vi "Do_Multical.vi"(7 "Rig Name":string, 9 "Rig Gas Selector Ch":T1[](array[typedef]) {"Duty" format="%.0b"; "D" format="%#_5g"; "C" format="%#_5g"; "B" format="%#_5g"; "A" format="%#_5g"}, 10 "Cal Gas Selection":string[](array[string]), 11 "Calib Filepaths":path[](array[path])) -> (2 "Cal Data":dbl[][](array[numeric]), 3 "Ref Data":dbl[](array[numeric]))   [LabVIEW 2015]
doc: "Step through the Calibration Procedure:\n1. Prompt user to connect appropriate / expected Cal Gas\n2. Update \"Gas Selector\" ADAM Ch which points to the current Cal Gas ADAM Ch\n3. Wait for sample to reach FID and settle\n4. Get a calibration data point for each FID"
uses:
  ADAM Client/Sub VIs/ADAM Controls/Ch_description_ADAM.ctl
  ADAM Client/Sub VIs/ADAM Controls/Module_type_ADAM.ctl
  ADAM Client/Sub VIs/ADAM Controls/Function_ADAM.ctl
  ADAM Client/Sub VIs/ADAM Controls/Channel_State.ctl
  ADAM Client/Sub VIs/ADAM Controls/Calib_type_ADAM.ctl
  ADAM Client/Sub VIs/ADAM Controls/Address.ctl
panel:
  in  "Tab Control":enum32{"Input", "Output"}(tab)
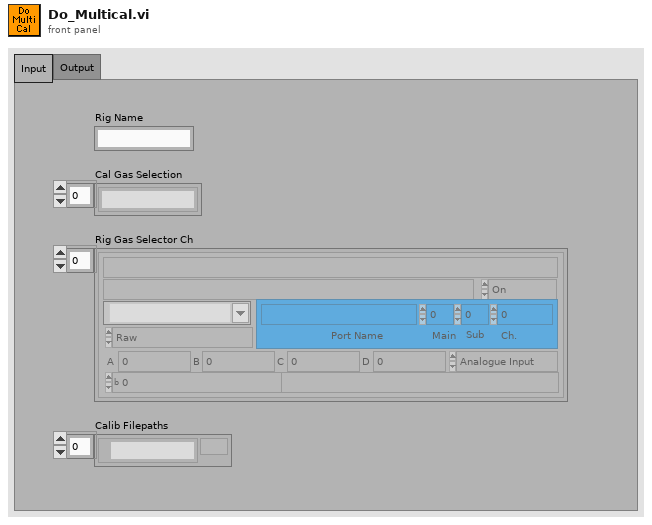
[diagram p1: front panel]
types:
  T1 = typedef "Ch_description_ADAM.ctl" = cluster{"Ch Name":string, "Type":T2, "Function":T3, "Ch State":T4, "Calibration type":T5, "A":dbl, "B":dbl, "C":dbl, "D":dbl, "Comments":string, "Address":T6, "String":string, "Duty":u16}
  T2 = typedef "Module_type_ADAM.ctl" = string
  T3 = typedef "Function_ADAM.ctl" = enum16{"Analogue Input", "Digital Input", "Event counter", "Event rate", "Analogue Output", "Digital Output", "Relay Output"}
  T4 = typedef "Channel_State.ctl" = enum16{"On", "Off", "Always On", "Always Off"}
  T5 = typedef "Calib_type_ADAM.ctl" = enum16{"Raw", "Bx + A", "Cx^2 + Bx + A", "Dx^3 + Cx^2 + Bx + A", "In Band", "Hi-Tec Q", "Hi-Tec M_dot", "Text"}
  T6 = typedef "Address.ctl" = cluster{"Main":i32, "Ch.":i32, "Sub":i32, "Port Name":string}
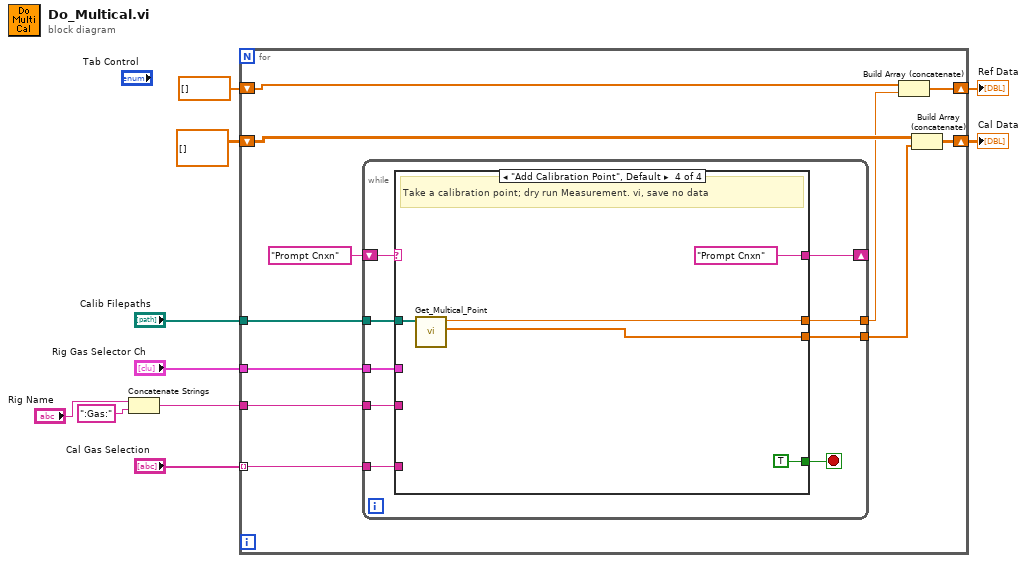
[diagram p0: block diagram]
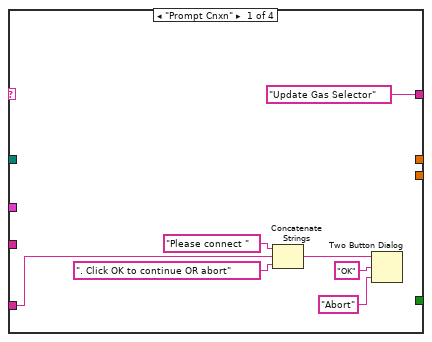
[diagram p2: hidden frame]
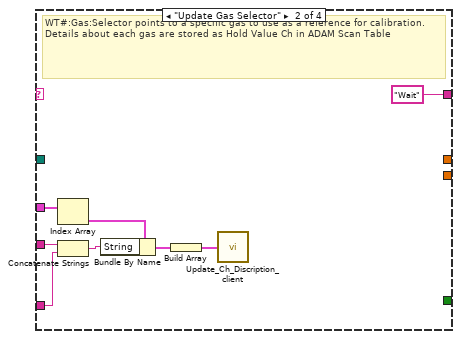
[diagram p3: hidden frame]
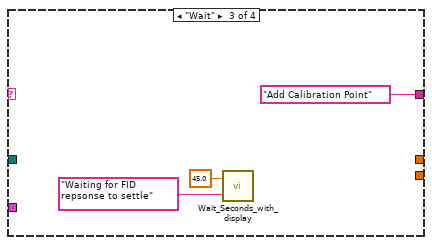
[diagram p4: hidden frame]
diagram:
  n1 = Concatenate Strings("Rig Name", ":Gas:") -> (w5:string)
  n2 = for {
    tunnel: "Cal Gas Selection" -> [w21] mode=indexing
    tunnel: "Rig Gas Selector Ch" -> [w19]
    tunnel: w5 -> [w18]
    tunnel: "Calib Filepaths" -> [w17]
    shift-right: [w15] -> w3
    shift-left: dbl[][] [] -> [w14]
    shift-right: [w12] -> w1
    shift-left: dbl[] [] -> [w11]
    n3 = while {
      tunnel: w21 -> [w30]
      shift-right: [w28] -> _
      shift-left: "Prompt Cnxn" -> [w29]
      tunnel: w19 -> [w27]
      tunnel: w18 -> [w26]
      tunnel: w17 -> [w25]
      tunnel: [w23] -> w16
      tunnel: [w22] -> w13
      stop <- w24 stop-if-true
      n4 = case shown="\"Add Calibration Point\", Default" w29 {
        tunnel: w30 -> [w36 w39 _ _]
        tunnel: ["Update Gas Selector" "Wait" "Add Calibration Point" "Prompt Cnxn"] -> w28
        tunnel: w27 -> [_ w42 _ _]
        tunnel: w26 -> [_ w40 _ _]
        tunnel: w25 -> [_ _ _ w53]
        tunnel: [_ _ _ TRUE] -> w24
        tunnel: [_ _ _ w50] -> w23
        tunnel: [_ _ _ w49] -> w22
        frame "Prompt Cnxn" {
          n5 = Concatenate Strings("Please connect " ("message"), w36, ". Click OK to continue OR abort" ("string")) -> (w32:string)
          n6 = Two Button Dialog(message=w32, 1:"Abort" ("F button name (\"Cancel\")"), 2:"OK" ("T button name (\"OK\")")) -> ()  [unwired: 1 out]
        }
        frame "Update Gas Selector" {
          # "WT#:Gas:Selector points to a specific gas to use as a reference for calibration. Details about each gas are stored as Hold Value Ch in ADAM Scan Table"
          n7 = Index Array(array=w42) -> (element=w43:T1)  [unwired: 1 in]
          n8 = Concatenate Strings(w40, w39) -> (w38:string)
          n9 = Bundle By Name(cluster=w43, "String"=w38) -> (w44:T1)
          n10 = Build Array(w44) -> (w45:T1[])
          n11 = call "Update_Ch_Discription_client.vi"("Channels to update In"=w45) -> ()  [unwired: 1 in]
        }
        frame "Wait" {
          n12 = call "Wait_Seconds_with_display.vi"("Message"="Waiting for FID repsonse to settle", "Seconds to wait"=45.0) -> ()  [unwired: 1 in, 1 out]
        }
        frame "Add Calibration Point", Default {
          # "Take a calibration point; dry run Measurement. vi, save no data"
          n13 = call "Get_Multical_Point.vi"("Calib Fnames OUT"=w53) -> ("Cal Points"=w50:dbl[], "Ref Val"=w49:dbl)  [unwired: 9 in]
        }
      }
    }
    n14 = Build Array (concatenate)(w11, w13) -> (w12:dbl[])
    n15 = Build Array (concatenate)(w14, w16) -> (w15:dbl[][])
  }
  "Cal Data" <- w3
  "Ref Data" <- w1
